vi "N-Close.vi"(8 "error in":errorcluster, 11 "Q Name":string) -> (0 "error out":errorcluster)   [LabVIEW 2016]
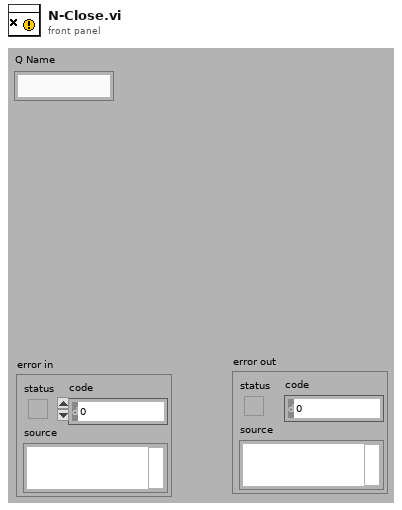
[diagram p1: front panel]
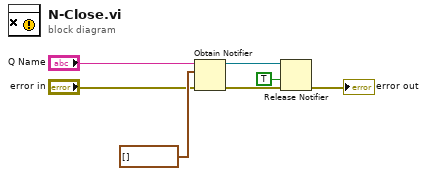
[diagram p0: block diagram]
diagram:
  n1 = Obtain Notifier(name (unnamed)="Q Name", notification data type=waveform(dbl)[] [] ("Waveform"), error in (no error)="error in") -> (notifier out=w3:refnum<notifier>, error out=w4:errorcluster)  [unwired: 1 in, 1 out]
  n2 = Release Notifier(notifier=w3, force destroy? (F)=TRUE, error in (no error)=w4) -> (error out=→"error out":errorcluster)  [unwired: 2 out]
